vi "String Included Different Case.vi"() -> ()   [LabVIEW 2017, in "Assertions.Tests.lvlib" / "Assert String Contains String Ignoring Case.lvlib"]
uses:
  Assert String Contains String Ignoring Case.lvlib
  src/Transparent Assertions/Assertions/Assertions.lvlib
panel:
  out "error out":errorcluster
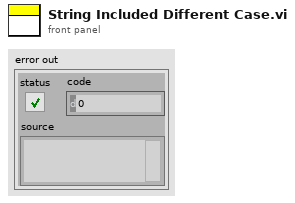
[diagram p1: front panel]
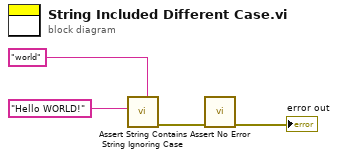
[diagram p0: block diagram]
diagram:
  n1 = call "Assert String Contains String Ignoring Case.vi"("Needle"="world", "Haystack"="Hello WORLD!") -> ("error out"=w2:errorcluster)  [unwired: 9 in]
  n2 = call "Assert No Error.vi"("error in (no error)"=w2) -> ("error out"=→"error out":errorcluster)  [unwired: 10 in]
